vi "Save Graph Data.vi"(0 "refnum in":refnum<file>, 1 "Save Data Enable":bool, 5 "Optic Sensor Data":dbl, 7 "Degrees":dbl, 11 "error in":errorcluster) -> (4 "refnum out":refnum<file>, 15 "error out":errorcluster)   [LabVIEW 2025, in "Control de MaP.lvlib"]
uses:
  Control de MaP.lvlib
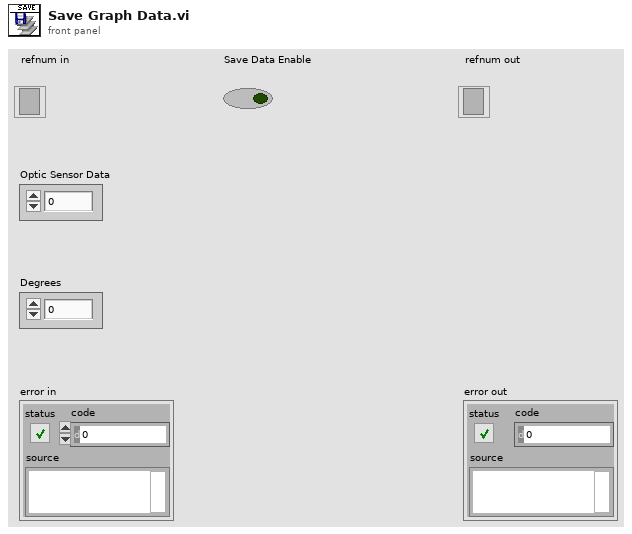
[diagram p1: front panel]
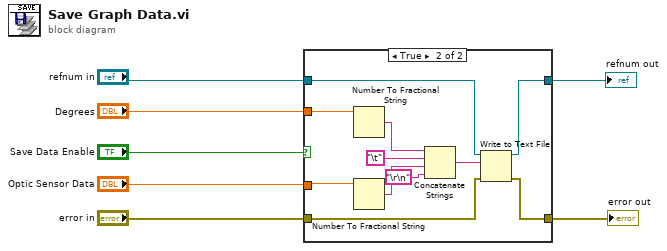
[diagram p0: block diagram]
diagram:
  n1 = case shown="True" "Save Data Enable" {
    tunnel: "refnum in" -> [w8 w20]
    tunnel: "Optic Sensor Data" -> [_ w19]
    tunnel: "Degrees" -> [_ w18]
    tunnel: "error in" -> [w9 w15]
    tunnel: [w9 w14] -> w4
    tunnel: [w8 w13] -> w3
    frame False {
    }
    frame True {
      n2 = Number To Fractional String(number=w18) -> (F-format string=w17:string)  [unwired: 3 in]
      n3 = Number To Fractional String(number=w19) -> (F-format string=w16:string)  [unwired: 3 in]
      n4 = Concatenate Strings(w17, "\t", w16, "\r\n") -> (w12:string)
      n5 = Write to Text File(file (use dialog)=w20, text=w12, error in=w15) -> (refnum out=w13:refnum<file>, error out=w14:errorcluster)  [unwired: 1 in, 1 out]
    }
  }
  "error out" <- w4
  "refnum out" <- w3
